vi "Create Backup.vi"(8 "error in":errorcluster, 11 "array of devices":T1) -> (0 "error out":errorcluster)   [LabVIEW 2016]
uses:
  Array Device Info.ctl
  Device Info.ctl
  Globals.vi
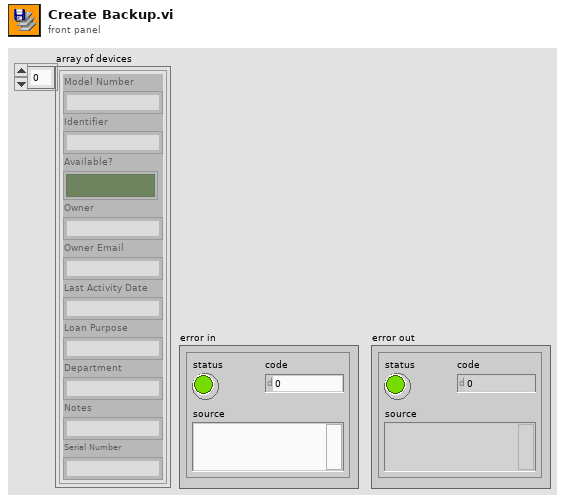
[diagram p1: front panel]
types:
  T1 = typedef "Array Device Info.ctl" = T2[]
  T2 = typedef "Device Info.ctl" = cluster{"Model Number":string, "Identifier":string, "Available?":bool, "Owner":string, "Owner Email":string, "Last Activity Date":string, "Loan Purpose":string, "Department":string, "Notes":string, "Serial Number":string}
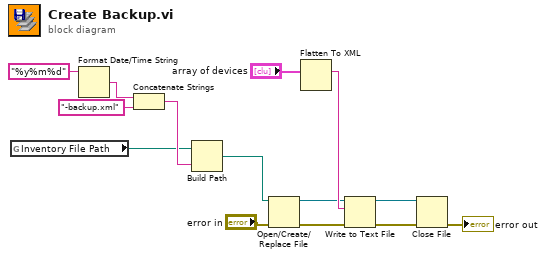
[diagram p0: block diagram]
diagram:
  n1 = global read "Globals.vi" "Inventory File Path"() -> (w2:path)
  n2 = Format Date/Time String(time format string (%c)="%y%m%d") -> (date/time string=w5:string)  [unwired: 2 in]
  n3 = Concatenate Strings(w5, "-backup.xml" ("string")) -> (w3:string)
  n4 = Build Path(base path=w2, name or relative path=w3) -> (appended path=w1:path)
  n5 = Open/Create/Replace File(file path (use dialog)=w1, error in="error in") -> (refnum out=w10:refnum<file>, error out=w12:errorcluster)  [unwired: 4 in, 1 out]
  n6 = Flatten To XML(anything="array of devices") -> (xml string=w14:string)
  n7 = Write to Text File(file (use dialog)=w10, text=w14, error in=w12) -> (refnum out=w11:refnum<file>, error out=w13:errorcluster)  [unwired: 1 in, 1 out]
  n8 = Close File(refnum=w11, error in=w13) -> (error out=→"error out":errorcluster)  [unwired: 1 out]
